vi "dfd_MA_Wrapper.vi"(11 "input data":fxp<+/-,16,16>) -> (3 "output data":fxp<+/-,32,2> format="%.31g")   [LabVIEW 2017]
uses:
  <vilib>/rvi/Emulation/niFpgaGetClockAttributes.vi
  <vilib>/rvi/Emulation/niFpgaSctlEmulationGetInTimedLoop.vi
  <vilib>/rvi/Emulation/niFpgaEmulationReportErrorSimple.vi
  <vilib>/rvi/Emulation/niFpgaCriticalErrorInLSC.vi
panel:
  in  "output valid":bool
  in  "data output":fxp<+/-,32,2> format="%.31g"
  out "valid input":bool
  out "data input":fxp<+/-,16,16>
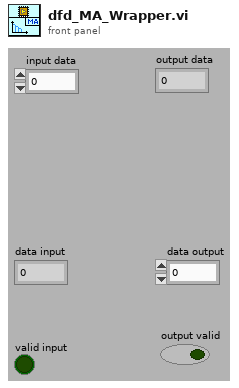
[diagram p1: front panel]
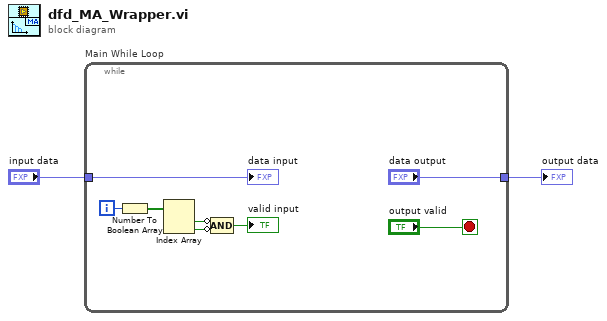
[diagram p0: block diagram]
diagram:
  n1 = while "Main While Loop" {
    tunnel: ["data output"] -> w2
    tunnel: "input data" -> [w8]
    i -> [w7]
    stop <- "output valid" stop-if-true
    n2 = Number To Boolean Array(number=w7) -> (Boolean array=w6:bool[])
    n3 = Index Array(array=w6) -> (element #1=w5:bool, element #2=w4:bool)  [unwired: 2 in]
    n4 = Compound Arithmetic op=AND(invert w5, invert w4) -> (→"valid input":bool)
    "data input" <- w8
  }
  "output data" <- w2
